vi "Get Channel Name Append String.vi"(8 "error in (no error)":errorcluster, 11 "Plugin In":refnum<class "Sequencer with Output Values.lvclass">) -> (0 "error out":errorcluster, 2 "Channel Append String":string, 3 "Plugin Out":refnum<class "Sequencer with Output Values.lvclass">)   [LabVIEW 2020, in "Sequencer with Output Values.lvlib" / "Sequencer with Output Values.lvclass"]
uses:
  Sequencer with Output Values.lvclass
  C:/Program Files/National Instruments/LabVIEW 2024/vi.lib/FlexLogger/SDK/PluginSDK.lvlibp/PEFClasses/SDK/Plugin/Plugin.lvclass
  <vilib>/FlexLogger/SDK/PluginSDK.lvlibp/PEFClasses/SDK/Producer Channel/Producer Channel.lvclass
  C:/Program Files/National Instruments/LabVIEW 2024/vi.lib/FlexLogger/SDK/PluginSDK.lvlibp/PEFClasses/SDK/Channel/Channel.lvclass
  <vilib>/FlexLogger/SDK/PluginSDK.lvlibp/PEFClasses/SDK/Plugin/Get Valid Producer Channels.vi
  Global Strings.vi
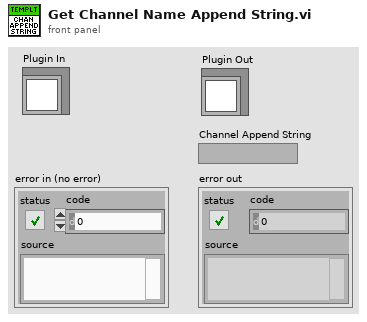
[diagram p1: front panel]
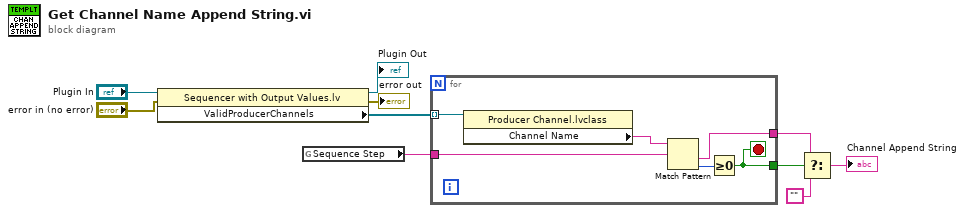
[diagram p0: block diagram]
diagram:
  n1 = property class="Sequencer with Output Values.lv"(reference="Plugin In", error in="error in (no error)") -> (reference out=→"Plugin Out":refnum<class "Sequencer with Output Values.lvclass">, error out=→"error out":errorcluster, "ValidProducerChannels"=w4:refnum<class "Producer Channel.lvclass">[])
  n2 = global read "Global Strings.vi" "Sequence Step"() -> (w5:string)
  n3 = for {
    tunnel: w4 -> [w16] mode=indexing
    tunnel: w5 -> [w13]
    tunnel: [w12] -> w2
    tunnel: [w15] -> w3
    stop <- w15 stop-if-true
    n4 = property class="Producer Channel.lvclass"(reference=w16) -> ("Channel Name"=w14:string)  [unwired: 1 in, 2 out]
    n5 = Match Pattern(string=w14, regular expression=w13) -> (after substring=w12:string, offset past match=w11:i32)  [unwired: 1 in, 2 out]
    n6 = Greater Or Equal To 0?(x=w11) -> (x >= 0?=w15:bool)
  }
  n7 = Select(t=w2, s=w3, f="") -> (s? t:f=→"Channel Append String":string)
